vi "AcquireSingalsF2.vi"(8 "error in (no error)":errorcluster, 9 "Stop Button":bool, 10 "Num of samp":i32=1000, 11 "rate [Hz]":dbl=2000.0) -> (0 "error out":errorcluster, 2 "Waveform Chart":dynamicdata(graph))   [LabVIEW 2021]
panel:
  out "stopped":bool
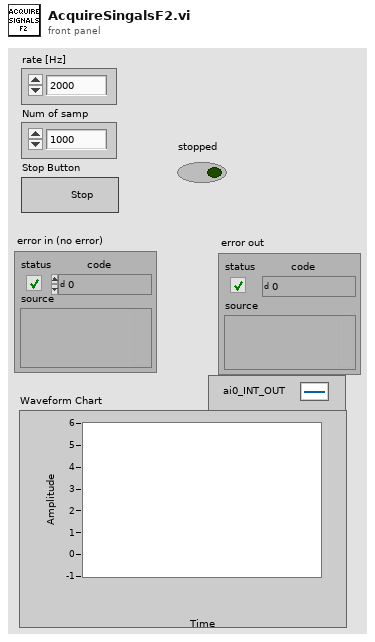
[diagram p1: front panel]
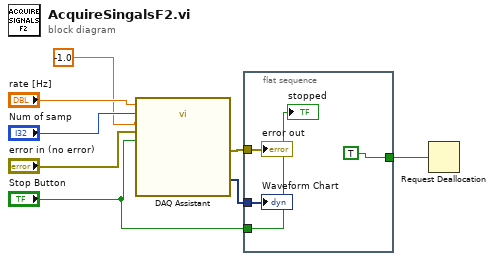
[diagram p0: block diagram]
diagram:
  n1 = call "DAQ Assistant"("rate"="rate [Hz]", "number of samples"="Num of samp", "timeout (s)"=-1.0, "error in"="error in (no error)", "stop (T)"="Stop Button") -> ("data"=w4:dynamicdata, "error out"=w5:errorcluster)  [unwired: 12 in, 1 out]
  n2 = flat-sequence {
    tunnel: w5 -> [w12]
    tunnel: w4 -> [w11]
    tunnel: [TRUE] -> w3
    tunnel: "Stop Button" -> [w9]
    frame #0 {
      "error out" <- w12
      "stopped" <- w9
      "Waveform Chart" <- w11
    }
  }
  n3 = Request Deallocation(w3) -> ()
